vi "Register VI Ref.vi"(8 "error in (no error)":errorcluster, 10 "VI ref":refnum<vi>, 11 "Viewable Actor in":refnum<class "Viewable Actor.lvclass">) -> (0 "error out":errorcluster, 3 "Viewable Actor out":refnum<class "Viewable Actor.lvclass">)   [LabVIEW 2014, in "Viewable Actor.lvlib" / "Viewable Actor.lvclass"]
uses:
  Viewable Actor.lvclass
  Viewable Actor.lvclass/Viewable Actor.ctl
  ActorMeter/ActorMeter Messages/Set Child VI Ref Msg/Set Child VI Ref Msg.lvclass/Set Child VI Ref Msg.ctl
  <vilib>/ActorFramework/Message Enqueuer/Message Enqueuer.lvclass/Message Enqueuer.ctl
  <vilib>/ActorFramework/Message Enqueuer/Enqueue.vi
  <vilib>/ActorFramework/Message Priority Queue/Priority Enqueue.vi
  <vilib>/ActorFramework/Message Enqueuer/Message Enqueuer.lvclass
  ActorMeter/ActorMeter Messages/Set Child VI Ref Msg/Set Child VI Ref Msg.lvclass
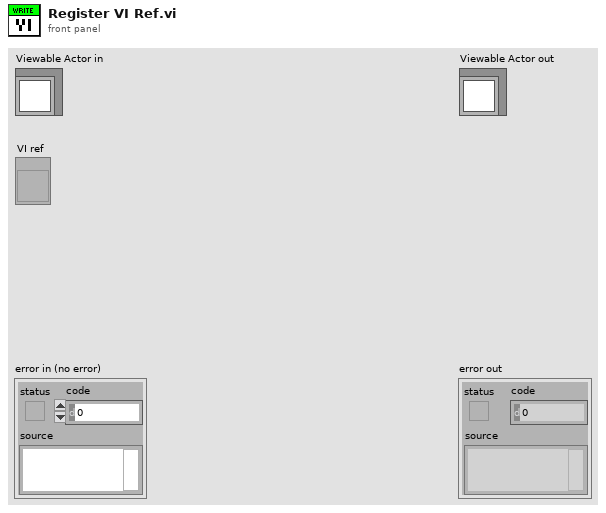
[diagram p1: front panel]
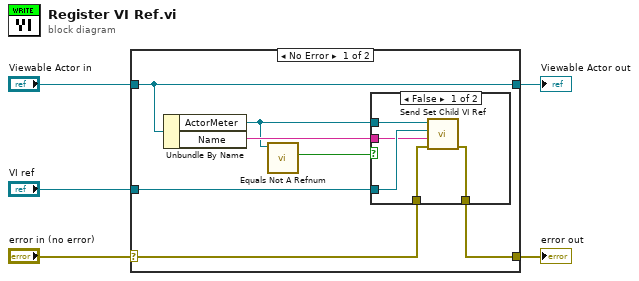
[diagram p0: block diagram]
diagram:
  n1 = case shown="No Error" "error in (no error)" {
    selector: "error in (no error)" -> [w9 w19]
    tunnel: [w8 w19] -> w4
    tunnel: [w12 w20] -> w2
    tunnel: "Viewable Actor in" -> [w12 w20]
    tunnel: "VI ref" -> [w11 _]
    frame No Error {
      n2 = Unbundle By Name(w12) -> ("ActorMeter"=w7:refnum<class "Message Enqueuer.lvclass">, "Name"=w10:string)
      n3 = call <vilib>:"Equals Not A Refnum.vi"("Message Enqueuer"=w7) -> ("Not a refnum?"=w6:bool)  [unwired: 10 in]
      n4 = case shown="False" w6 {
        tunnel: w7 -> [w17 _]
        tunnel: w11 -> [w16 _]
        tunnel: w10 -> [w15 _]
        tunnel: w9 -> [w14 w18]
        tunnel: [w13 w18] -> w8
        frame False {
          n5 = call "Send Set Child VI Ref.vi"("error in (no error)"=w14, "Name"=w15, "VI ref"=w16, "Message Enqueuer"=w17) -> ("error out"=w13:errorcluster)  [unwired: 6 in, 1 out]
        }
        frame True {
        }
      }
    }
    frame Error {
    }
  }
  "error out" <- w4
  "Viewable Actor out" <- w2
